vi "GetControls.vi"(6 "error in":errorcluster, 9 "Cluster in":refnum<class "Cluster.lvclass">) -> (0 "error out":errorcluster, 3 "Cluster in":refnum<class "Cluster.lvclass">, 4 "controls":cluster{"controls":i32[], "decorations":i32[]})   [LabVIEW 2014, in "Raspberry Pi Compatible Compiler for LabVIEW.lvlib" / "Cluster.lvclass"]
uses:
  Cluster.lvclass
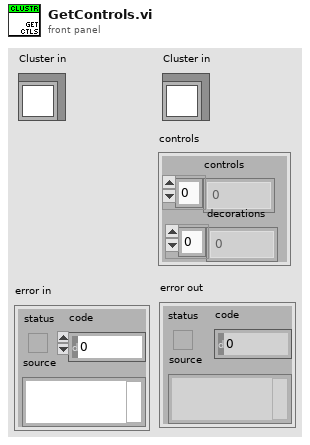
[diagram p1: front panel]
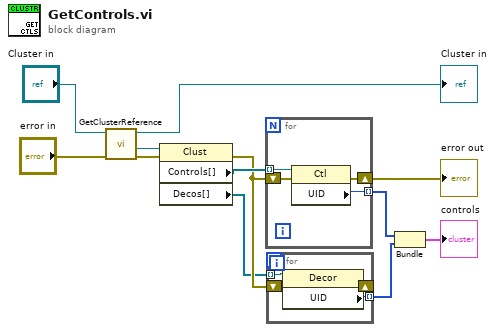
[diagram p0: block diagram]
diagram:
  n1 = call "GetClusterReference.vi"("error in"="error in", "Cluster in"="Cluster in") -> ("error out"=w2:errorcluster, "cluster reference"=w3:refnum<vi>, "Cluster out"=→"Cluster in":refnum<class "Cluster.lvclass">)  [unwired: 7 in]
  n2 = property class="Clust"(reference=w3, error in=w2) -> (error out=w6:errorcluster, "Controls[]"=w8:refnum<vi>[], "Decos[]"=w5:refnum<vi>[])  [unwired: 1 out]
  n3 = for {
    tunnel: w8 -> [w15] mode=indexing
    shift-right: [w14] -> w9
    shift-left: w6 -> [w16]
    tunnel: [w13] -> w7 mode=indexing
    n4 = property class="Ctl"(reference=w15, error in=w16) -> (error out=w14:errorcluster, "UID"=w13:i32)  [unwired: 1 out]
  }
  "error out" <- w9
  n5 = for {
    tunnel: w5 -> [w19] mode=indexing
    shift-right: [w18] -> _
    shift-left: w6 -> [w20]
    tunnel: [w17] -> w4 mode=indexing
    n6 = property class="Decor"(reference=w19, error in=w20) -> (error out=w18:errorcluster, "UID"=w17:i32)  [unwired: 1 out]
  }
  n7 = Bundle(w7, w4) -> (→"controls":cluster{i32[], i32[]})  [unwired: 1 in]
